vi "NB_ReadWriteAttribute_IPE.vi"(0 "object in":refnum<class "NativeBaseTemplate.lvclass">, 5 "Error In":errorcluster) -> (14 "object out":refnum<class "NativeBaseTemplate.lvclass">, 19 "Error Out":errorcluster)   [LabVIEW 2020, in "NativeBaseTemplate.lvclass"]
uses:
  <resource>/Framework/Providers/Open_GDS/ClassProviders/Provider_LvNativeClass/Templates/NativeBaseTemplate/NativeBaseTemplate.lvclass
  <resource>/Framework/Providers/Open_GDS/ClassProviders/Provider_LvNativeClass/Templates/NativeBaseTemplate/NativeBaseTemplate.lvclass/NativeBaseTemplate.ctl
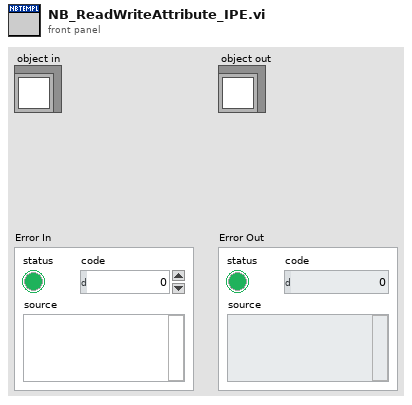
[diagram p1: front panel]
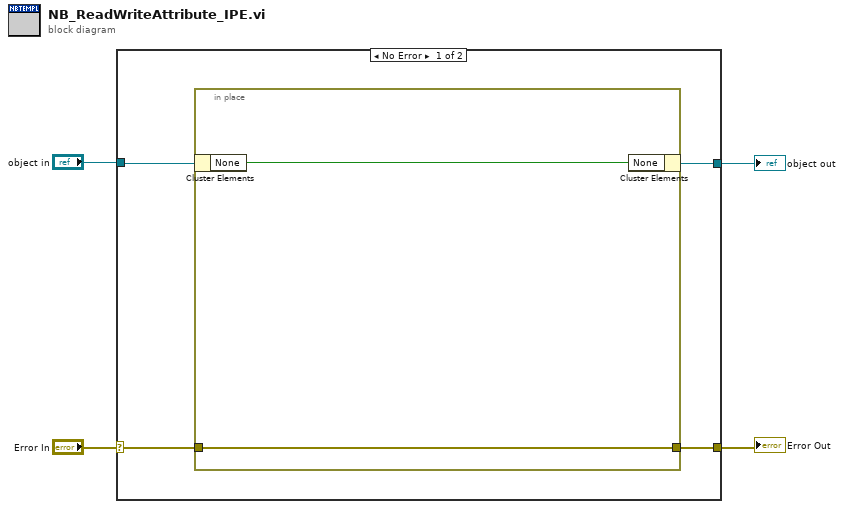
[diagram p0: block diagram]
diagram:
  n1 = case shown="No Error" "Error In" {
    selector: "Error In" -> [w5 w12]
    tunnel: [w6 w12] -> w3
    tunnel: [w7 w11] -> w1
    tunnel: "object in" -> [w8 w11]
    frame No Error {
      n2 = in-place {
        in-place-border: [w9] -> w6
        in-place-border: w5 -> [w9]
        n3 = in-place-cluster #1(w8) -> ("None"=w10:bool)
        n4 = in-place-cluster #1("None"=w10) -> (w7:refnum<class "NativeBaseTemplate.lvclass">)
      }
    }
    frame Error {
    }
  }
  "Error Out" <- w3
  "object out" <- w1
